vi "Write commandFactory.vi"(10 "commandFactory":refnum<class "ICommandFactory.lvclass">, 11 "DataListenerThisComponent in":refnum<class "DataListenerThisComponent.lvclass">) -> (3 "DataListenerThisComponent out":refnum<class "DataListenerThisComponent.lvclass">)   [LabVIEW 2015, in "DataListenerThisComponent.lvclass"]
uses:
  DataListenerThisComponent.lvclass
  ICommandFactory/ICommandFactory.lvclass
  DataListenerThisComponent.lvclass/DataListenerThisComponent.ctl
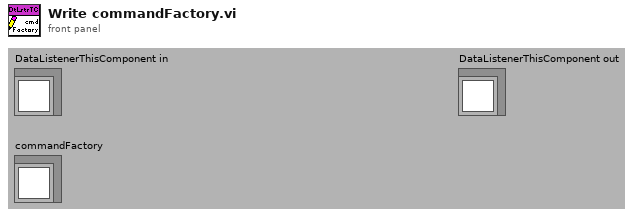
[diagram p1: front panel]
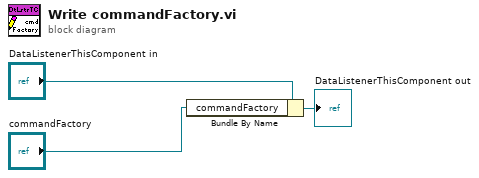
[diagram p0: block diagram]
diagram:
  n1 = Bundle By Name(cluster="DataListenerThisComponent in", "commandFactory"="commandFactory") -> (→"DataListenerThisComponent out":refnum<class "DataListenerThisComponent.lvclass">)
